vi "From JSON.vi"(8 "error in (no error)":errorcluster, 10 "JSON":string, 11 "Type in":refnum<class "Abs_String 1D.lvclass">) -> (0 "error out":errorcluster, 3 "Type out":refnum<class "Abs_String 1D.lvclass">)   [LabVIEW 2021, in "Abs_String 1D.lvclass"]
uses:
  Abs_String 1D.lvclass
  C:/Program Files (x86)/National Instruments/LabVIEW 2021/vi.lib/TSA/Abstract Data Classes/Abs_Types/Type/Abs_Type.lvclass
  84995497-0203-4e81-9b13-3fa8bc9bad62.vi
  <vilib>/JDP Science/JSONtext/Find Item.vi
  <vilib>/JDP Science/JSONtext/Next JSON Value.vi
  <vilib>/JDP Science/JSONtext/String Subset.vi
  <vilib>/JDP Science/JSONtext/Parsing/Advance past next JSON Value (inlined COPY).vi
  <vilib>/JDP Science/JSONtext/Parsing/Advance past whitespace.vi
  <vilib>/JDP Science/JSONtext/Parsing/Advance past String.vi
  <vilib>/JDP Science/JSONtext/Parsing/Advance past Number.vi
  <vilib>/JDP Science/JSONtext/Parsing/Advance past Line Ending.vi
  <vilib>/Utility/LVClass/Get LV Class Name.vi
  <vilib>/JDP Science/JSONtext/Parsing/Parse Full Path or Item Name.vi
  <vilib>/JDP Science/JSONtext/Parsing/Advance past Array.vi
  <vilib>/JDP Science/JSONtext/Parsing/Advance past Object.vi
  <vilib>/JDP Science/JSONtext/support/Error Cluster From Code.vi
  <vilib>/JDP Science/JSONtext/Offset/Find Item Locations by Path.vi
  <vilib>/JDP Science/JSONtext/JSON text to Variant.vi
  <vilib>/JDP Science/JSONtext/LVClass Serializer/JSONtext LVClass Serializer.lvclass
  Array 1D/Abs_Array1D.lvclass
  Type/Abs_Type.lvclass
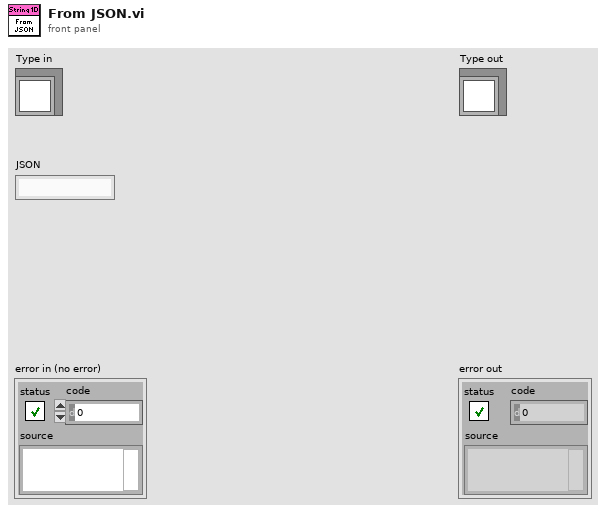
[diagram p1: front panel]
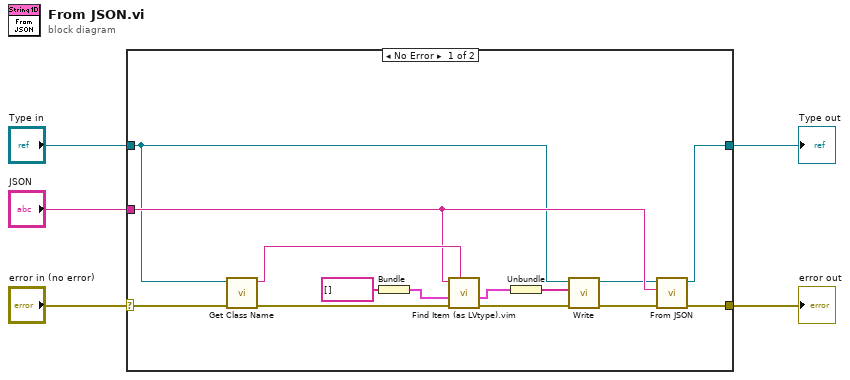
[diagram p0: block diagram]
diagram:
  n1 = case shown="No Error" "error in (no error)" {
    selector: "error in (no error)" -> [w15 w20]
    tunnel: [w19 w20] -> w2
    tunnel: [w18 w21] -> w1
    tunnel: "JSON" -> [w13 _]
    tunnel: "Type in" -> [w7 w21]
    frame No Error {
      n2 = call "Get Class Name.vi"("error in (no error)"=w15, "Abs_Type in"=w7) -> ("error out"=w12:errorcluster, "class name"=w14:string)  [unwired: 8 in]
      n3 = Bundle(string[] []) -> (w16:cluster{string[]})  [unwired: 1 in]
      n4 = call "Find Item (as LVtype).vim"("$Path or Item Name"=w14, "error in (no error)"=w12, "Data Type and Default Value"=w16, "JSON"=w13) -> ("error out"=w11:errorcluster, "Data"=w17:cluster{string[]})  [unwired: 4 in, 2 out]
      n5 = Unbundle(w17) -> (w8:string[])
      n6 = call-dynamic "Write.vi"("error in (no error)"=w11, "Array"=w8, "Abs_String in"=w7) -> ("error out"=w10:errorcluster, "Abs_String out"=w9:refnum<class "Abs_String 1D.lvclass">)  [unwired: 7 in]
      n7 = call-parent "From JSON.vi"("error in (no error)"=w10, "JSON"=w13, "Type in"=w9) -> ("error out"=w19:errorcluster, "Type out"=w18:refnum<class "Abs_String 1D.lvclass">)  [unwired: 7 in]
    }
    frame Error {
    }
  }
  "error out" <- w2
  "Type out" <- w1
